vi "connectShMem.vi"(8 "error in (no error)":errorcluster, 11 "SalProcess in":refnum<class "SalProcess.lvclass">) -> (0 "error out":errorcluster, 2 "function return":i32, 3 "SalProcess out":refnum<class "SalProcess.lvclass">)   [LabVIEW 2018, in "SalProcess.lvclass"]
doc: "Connect the shared memory."
uses:
  SalProcess.lvclass
  SalProcess.lvclass/SalProcess.ctl
  LibReader/LibReader.lvclass
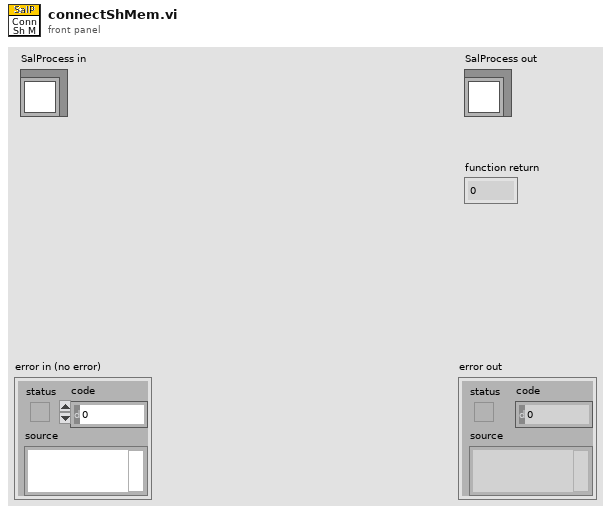
[diagram p1: front panel]
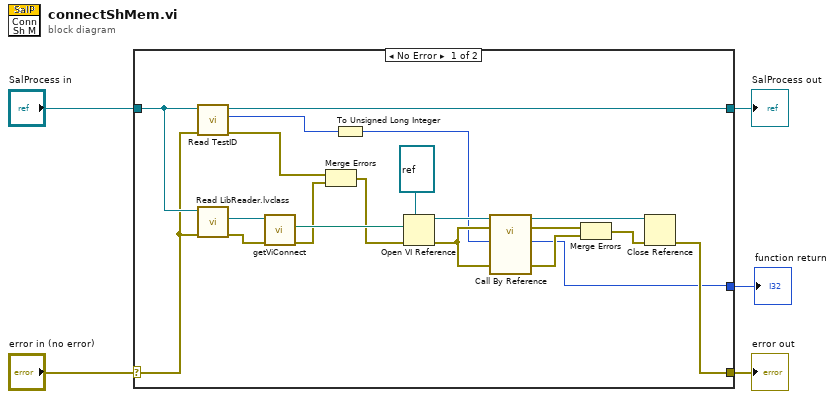
[diagram p0: block diagram]
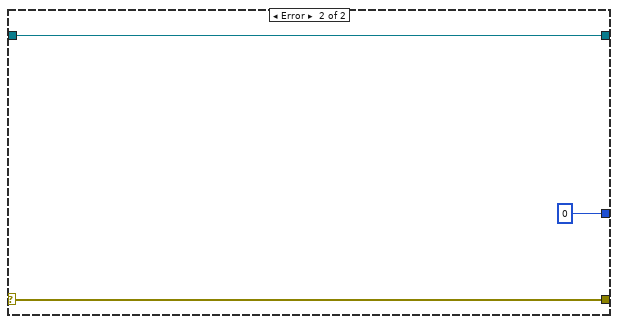
[diagram p2: hidden frame]
diagram:
  n1 = case shown="No Error" "error in (no error)" {
    selector: "error in (no error)" -> [w24 w28]
    tunnel: [w9 w28] -> w4
    tunnel: [w17 w27] -> w2
    tunnel: "SalProcess in" -> [w25 w27]
    tunnel: [w8 0 ("function return")] -> w1
    frame No Error {
      n2 = call "Read TestID.vi"("error in (no error)"=w24, "SalProcess in"=w25) -> ("error out"=w20:errorcluster, "TestID"=w7:i32, "SalProcess out"=w17:refnum<class "SalProcess.lvclass">)  [unwired: 7 in]
      n3 = call "Read LibReader.lvclass.vi"("error in (no error)"=w24, "SalProcess in"=w25) -> ("error out"=w22:errorcluster, "LibReader.lvclass"=w23:refnum<class "LibReader.lvclass">)  [unwired: 7 in, 1 out]
      n4 = call "getViConnect.vi"("error in (no error)"=w22, "LibReader in"=w23) -> ("error out"=w19:errorcluster, "pathViConnect"=w21:path)  [unwired: 7 in, 1 out]
      n5 = Merge Errors(w20, w19) -> (w18:errorcluster)
      n6 = To Unsigned Long Integer(number=w7) -> (unsigned 32bit integer=w6:u32)
      n7 = Open VI Reference(type specifier VI Refnum (for type only)=refnum<vi> refnum, vi path=w21, error in (no error)=w18) -> (vi reference=w15:refnum<vi>, error out=w14:errorcluster)  [unwired: 3 in]
      n8 = call-by-ref "?"(reference=w15, error in=w14, 8:"error in (no error)"=w14, "TestID"=w6) -> (reference out=w13:refnum<vi>, error out=w12:errorcluster, 0:"error out"=w11:errorcluster, "function return"=w8:i32)  [unwired: 8 in]
      n9 = Merge Errors(w12, w11) -> (w10:errorcluster)
      n10 = Close Reference(reference=w13, error in (no error)=w10) -> (error out=w9:errorcluster)
    }
    frame Error {
    }
  }
  "error out" <- w4
  "SalProcess out" <- w2
  "function return" <- w1
